vi "Configure Number of Points.vi"(8 "error in (no error)":errorcluster, 10 "Number of Point":i32, 11 "VNA-PNA in":refnum<class "VNA-PNA.lvclass">) -> (0 "error out":errorcluster, 3 "VNA-PNA out":refnum<class "VNA-PNA.lvclass">)   [LabVIEW 2020, in "VNA-PNA.lvclass"]
doc: "Configures the number of points in the sweep.\nThe number of points will be choosen to the nearest supported."
uses:
  VNA-PNA.lvclass
  C:/Sandbox/Git_Sandbox/WiSpry Test Framework source code (LV20)/WiSpry Test Framework/Instruments/Instrument.lvclass
  C:/Sandbox/Git_Sandbox/WiSpry Test Framework source code (LV20)/WiSpry Test Framework/Instruments/Vector Network Analyzer/Vector Network Analyzer.lvclass
  Instrument.lvclass/Instrument.ctl
  Vector Network Analyzer.lvclass/Vector Network Analyzer.ctl
  Instrument.lvclass
  Vector Network Analyzer.lvclass
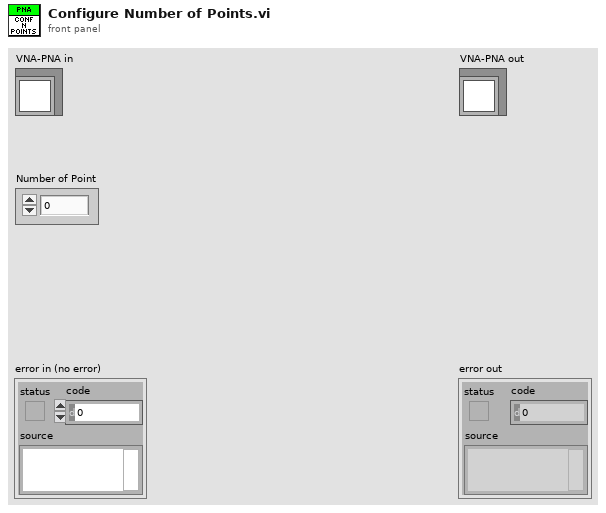
[diagram p1: front panel]
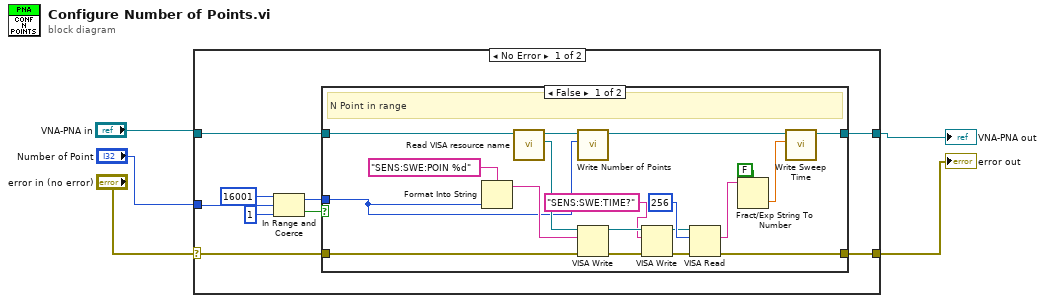
[diagram p0: block diagram]
diagram:
  n1 = case shown="No Error" "error in (no error)" {
    selector: "error in (no error)" -> [w8 w36]
    tunnel: "VNA-PNA in" -> [w9 w37]
    tunnel: "Number of Point" -> [w14 _]
    tunnel: [w7 w37] -> w2
    tunnel: [w6 w36] -> w1
    frame No Error {
      n2 = In Range and Coerce(upper limit=16001, x=w14, lower limit=1) -> (coerced(x)=w10:i32, In Range?=w11:bool)
      n3 = case shown="False" w11 {
        tunnel: w10 -> [w27 _]
        tunnel: w9 -> [w33 w35]
        tunnel: w8 -> [w29 w34]
        tunnel: [w24 w35] -> w7
        tunnel: [w20 w34] -> w6
        frame False {
          # "N Point in range"
          n4 = Format Into String(format string="SENS:SWE:POIN %d", w27) -> (resulting string=w31:string)  [unwired: 2 in, 1 out]
          n5 = call "Read VISA resource name.vi"("Instrument in"=w33) -> ("VISA resource name"=w30:refnum<visa-resource-name>, "Instrument out"=w28:refnum<class "VNA-PNA.lvclass">)  [unwired: 9 in]
          n6 = call "Write Number of Points.vi"("Number of Points"=w27, "Vector Network Analyzer in"=w28) -> ("Vector Network Analyzer out"=w25:refnum<class "VNA-PNA.lvclass">)  [unwired: 9 in]
          n7 = VISA Write(VISA resource name=w30, write buffer=w31, error in (no error)=w29) -> (VISA resource name out=w16:refnum<visa-resource-name>, error out=w17:errorcluster)  [unwired: 1 out]
          n8 = VISA Write(VISA resource name=w16, write buffer="SENS:SWE:TIME?", error in (no error)=w17) -> (VISA resource name out=w18:refnum<visa-resource-name>, error out=w19:errorcluster)  [unwired: 1 out]
          n9 = VISA Read(VISA resource name=w18, byte count=u32 256, error in (no error)=w19) -> (read buffer=w23:string, error out=w20:errorcluster)  [unwired: 2 out]
          n10 = Fract/Exp String To Number(use system decimal point (T)=FALSE, string=w23) -> (number=w21:dbl)  [unwired: 2 in, 1 out]
          n11 = call "Write Sweep Time.vi"("Sweep Time"=w21, "Vector Network Analyzer in"=w25) -> ("Vector Network Analyzer out"=w24:refnum<class "VNA-PNA.lvclass">)  [unwired: 9 in]
        }
        frame True {
          # "Add Error handler"
          # "Raise Error"
        }
      }
    }
    frame Error {
    }
  }
  "error out" <- w1
  "VNA-PNA out" <- w2
